vi "GetPrecision.vi"(8 "error in":errorcluster, 11 "RealMeasure in":refnum<class "RealMeasure.lvclass">) -> (0 "error out":errorcluster, 2 "Precision":u8=6, 3 "RealMeasure out":refnum<class "RealMeasure.lvclass">)   [LabVIEW 2021, in "ProligentXMLGenerator.lvlib" / "RealMeasure.lvclass"]
doc: "Defines the numeric precision of the measure value."
uses:
  RealMeasure.lvclass
  RealMeasure.lvclass/RealMeasure.ctl
  Base/UnsignedByte/UnsignedByte.lvclass
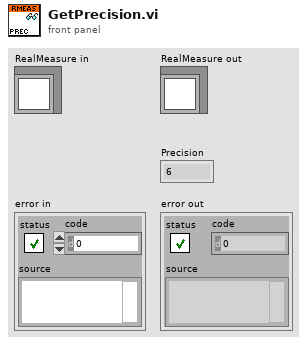
[diagram p1: front panel]
types:
  T1 = typedef "ProligentXMLGenerator.lvlib/RealMeasure.lvclass/Data.ctl" = cluster{"Value":refnum<class "Decimal.lvclass">, "Precision":refnum<class "UnsignedByte.lvclass">}
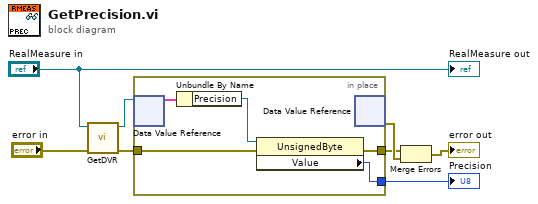
[diagram p0: block diagram]
diagram:
  n1 = call "GetDVR.vi"("error in"="error in", "RealMeasure"="RealMeasure in") -> ("error out"=w2:errorcluster, "DVRReference"=w7:refnum<data-value>)  [unwired: 8 in]
  n2 = in-place "In Place Element Structure" {
    in-place-border: [w12] -> w6
    in-place-border: w2 -> [w9]
    in-place-border: [w11] -> w1
    n3 = in-place-dvr #1(w7) -> (w13:T1)  [unwired: 1 out]
    n4 = Unbundle By Name(w13) -> ("Precision"=w10:refnum<class "UnsignedByte.lvclass">)
    n5 = property on="Property Node" class="UnsignedByte"(reference=w10, error in=w9) -> (error out=w11:errorcluster, "Value"=w12:u8)  [unwired: 1 out]
    n6 = in-place-dvr #1() -> (w8:errorcluster)  [unwired: 1 in, 1 out]
  }
  "Precision" <- w6
  n7 = Merge Errors(w1, w8) -> (→"error out":errorcluster)
  "RealMeasure out" <- "RealMeasure in"
